vi "HK Channel Write CVT Settings.vi"(8 "error in (no error)":errorcluster, 10 "CVT Settings":T1 {"Max Age" format="%<%H:%M:%S>t"}, 11 "HK Channel in":refnum<class "HK Table.lvclass">) -> (0 "error out":errorcluster, 3 "HK Channel out":refnum<class "HK Table.lvclass">)   [LabVIEW 2019, in "HK Table.lvclass"]
uses:
  HK Table.lvclass
  HK Current Value Table Settings.ctl
  HK Table.lvclass/HK Table.ctl
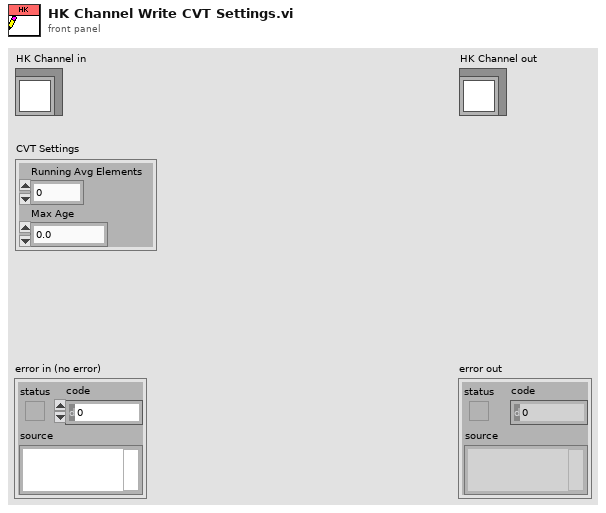
[diagram p1: front panel]
types:
  T1 = typedef "HK Table.lvclass/HK Current Value Table Settings.ctl" = cluster{"Running Avg Elements":i32, "Max Age":dbl}
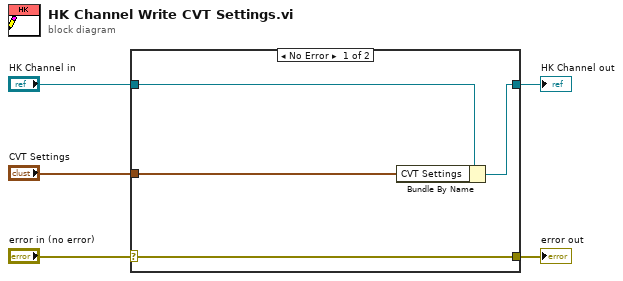
[diagram p0: block diagram]
diagram:
  n1 = case shown="No Error" "error in (no error)" {
    selector: "error in (no error)" -> [w9 w10]
    tunnel: [w9 w10] -> w4
    tunnel: [w7 w11] -> w2
    tunnel: "HK Channel in" -> [w8 w11]
    tunnel: "CVT Settings" -> [w6 _]
    frame No Error {
      n2 = Bundle By Name(cluster=w8, "CVT Settings"=w6) -> (w7:refnum<class "HK Table.lvclass">)
    }
    frame Error {
    }
  }
  "error out" <- w4
  "HK Channel out" <- w2
